vi "DSF.Engine.Memory.ObjectPool.Obtain Object.vi"(8 "error in (no error)":errorcluster, 9 "timeout ms (0)":i32 format="%d ms", 11 "ObjectPool in":refnum<class "DSF.Engine.Memory.ObjectPool.lvclass">) -> (0 "error out":errorcluster, 1 "timed out?":bool, 2 "ObjectPool Bundle":refnum<class "DSF.Engine.Memory.ObjectPool Bundle.lvclass">, 3 "ObjectPool out":refnum<class "DSF.Engine.Memory.ObjectPool.lvclass">)   [LabVIEW 2016, in "DSF.Engine.lvlib" / "DSF.Engine.Memory.ObjectPool.lvclass"]
uses:
  DSF.Engine.Memory.ObjectPool.lvclass
  DSF.Engine.Memory.ObjectPool Bundle.lvclass
  DSF.Engine.Memory.ObjectPool.lvclass/DSF.Engine.Memory.ObjectPool.ctl
  DSF.Engine.Memory.ObjectPool Bundle.lvclass/DSF.Engine.Memory.ObjectPool Bundle.ctl
  DSF.Engine.Memory.ObjectPool.Get Index FIFO.vi
  DSF.Engine.Memory.ObjectPool Bundle.Set Index.vi
  DSF.Engine.Memory.ObjectPool Bundle.Set Object.vi
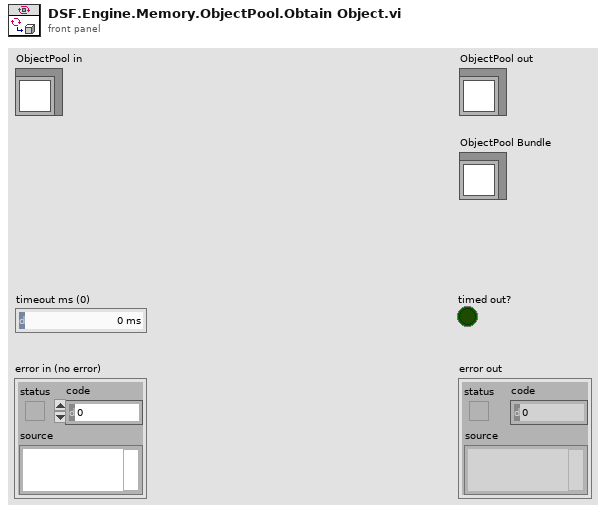
[diagram p1: front panel]
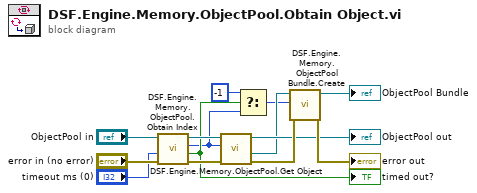
[diagram p0: block diagram]
diagram:
  n1 = call "DSF.Engine.Memory.ObjectPool.Obtain Index.vi"("error in (no error)"="error in (no error)", "timeout ms (0)"="timeout ms (0)", "ObjectPool in"="ObjectPool in") -> ("error out"=w10:errorcluster, "timed out?"=w4:bool, "index"=w1:i32, "ObjectPool out"=w11:refnum<class "DSF.Engine.Memory.ObjectPool.lvclass">)  [unwired: 5 in]
  "timed out?" <- w4
  n2 = call "DSF.Engine.Memory.ObjectPool.Get Object.vi"("error in (no error)"=w10, "index"=w1, "ObjectPool in"=w11) -> ("error out"=w9:errorcluster, "Object"=w6:refnum<class>, "ObjectPool out"=→"ObjectPool out":refnum<class "DSF.Engine.Memory.ObjectPool.lvclass">)  [unwired: 6 in]
  n3 = Select(t=-1 ("f"), s=w4, f=w1) -> (s? t:f=w3:i32)
  n4 = call "DSF.Engine.Memory.ObjectPool Bundle.Create.vi"("error in (no error)"=w9, "index"=w3, "Object"=w6) -> ("error out"=→"error out":errorcluster, "ObjectPool Bundle"=→"ObjectPool Bundle":refnum<class "DSF.Engine.Memory.ObjectPool Bundle.lvclass">)  [unwired: 7 in]
